vi "Release.vi"(8 "error in (no error)":errorcluster, 11 "Register JSON in":refnum<class "Register JSON.lvclass">) -> (0 "error out":errorcluster)   [LabVIEW 2020, in "wamplv.lvlib" / "Register JSON.lvclass"]
uses:
  Register JSON.lvclass
  Register JSON.lvclass/Register JSON.ctl
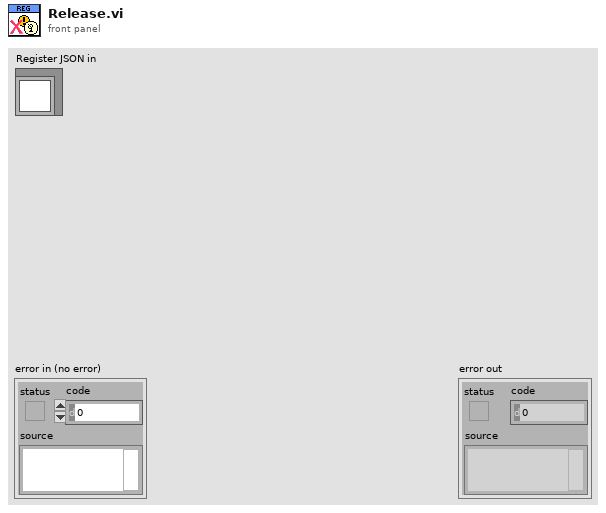
[diagram p1: front panel]
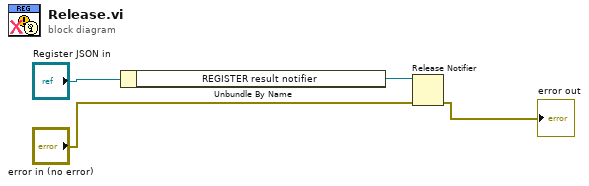
[diagram p0: block diagram]
diagram:
  n1 = Unbundle By Name("Register JSON in") -> ("REGISTER result notifier"=w3:refnum<notifier>)
  n2 = Release Notifier(notifier=w3, error in (no error)="error in (no error)") -> (error out=→"error out":errorcluster)  [unwired: 1 in, 2 out]
